vi "Refresh Skipfire Listbox.vi"(9 "ChannelNames":string[](array[string]), 10 "Skipfire Settings Array":T1[](array[typedef]), 11 "Skipfire Listbox Refnum":refnum<vi>) -> ()   [LabVIEW 2016, in "DCM System Explorer.lvlib"]
uses:
  DCM System Explorer.lvlib
  <vilib>/Powertrain Controls/Device Drivers/DCM/Skip Fire/RT/Skip Fire Setup.ctl
  <vilib>/Powertrain Controls/Device Drivers/DCM/Skip Fire/RT/DCM - RT - Skip Fire.lvlib
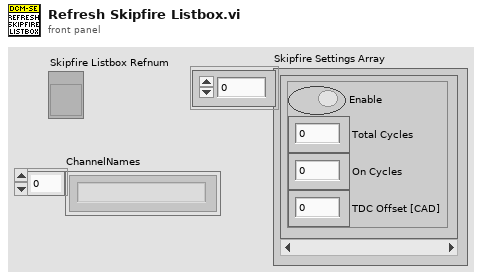
[diagram p1: front panel]
types:
  T1 = typedef "DCM - RT - Skip Fire.lvlib/Skip Fire Setup.ctl" = cluster{"Enable":bool, "Total Cycles":u8, "On Cycles":u8, "TDC Offset [CAD]":sgl}
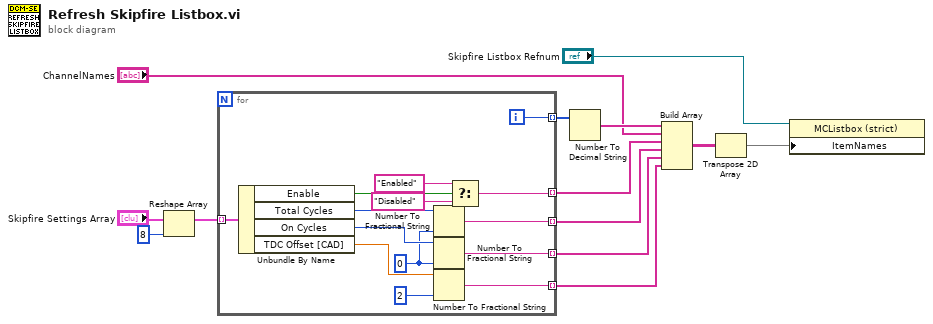
[diagram p0: block diagram]
diagram:
  n1 = Reshape Array("Skipfire Settings Array", 8) -> (w11:T1[])
  n2 = for {
    tunnel: w11 -> [w27] mode=indexing
    tunnel: [w15] -> w9 mode=indexing
    tunnel: [w23] -> w6 mode=indexing
    tunnel: [w21] -> w5 mode=indexing
    tunnel: [w17] -> w4 mode=indexing
    tunnel: [w16] -> w3 mode=indexing
    i -> [w15]
    w14 = i16 0 ("precision (6)")
    n3 = Unbundle By Name(w27) -> ("Enable"=w26:bool, "Total Cycles"=w22:u8, "On Cycles"=w19:u8, "TDC Offset [CAD]"=w18:sgl)
    n4 = Number To Fractional String(number=w22, precision (6)=w14) -> (F-format string=w21:string)  [unwired: 2 in]
    n5 = Number To Fractional String(number=w19, precision (6)=w14) -> (F-format string=w17:string)  [unwired: 2 in]
    n6 = Number To Fractional String(number=w18, precision (6)=i16 2) -> (F-format string=w16:string)  [unwired: 2 in]
    n7 = Select(t="Enabled", s=w26, f="Disabled") -> (s? t:f=w23:string)
  }
  n8 = Number To Decimal String(number=w9) -> (decimal integer string=w10:string[])  [unwired: 1 in]
  n9 = Build Array(w10, "ChannelNames", w6, w5, w4, w3) -> (w13:string[][])
  n10 = Transpose 2D Array(2D array=w13) -> (transposed array=w8:string[][])
  n11 = property on="Property Node" class="MCListbox (strict)"(reference="Skipfire Listbox Refnum", "ItemNames"=w8) -> ()  [unwired: 1 in, 2 out]
